vi "ATS9350_NPT_Scan.vi"(0 "Records per Buffer":u32=1000, 5 "Pt per A-line":u32=256, 7 "Total records number":u32, 9 "Numeric":dbl, 11 "Range":u32(ring)=10 items=["40 mV"=2, "100 mV"=5, "200 mV"=6, "400 mV"=7, "1 V"=10, "2 V"=11, "4 V"=12]) -> (4 "Device ID":u64)   [LabVIEW 2017]
panel:
  # "Connect proper signal to channel A before starting acquisition\n(e.g. 1Vpp 1kHz sine wave)"
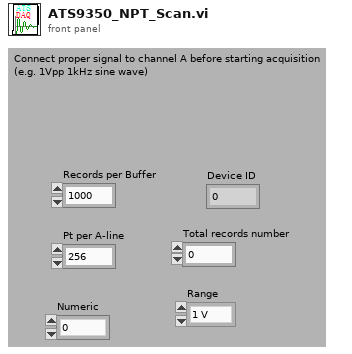
[diagram p1: front panel]
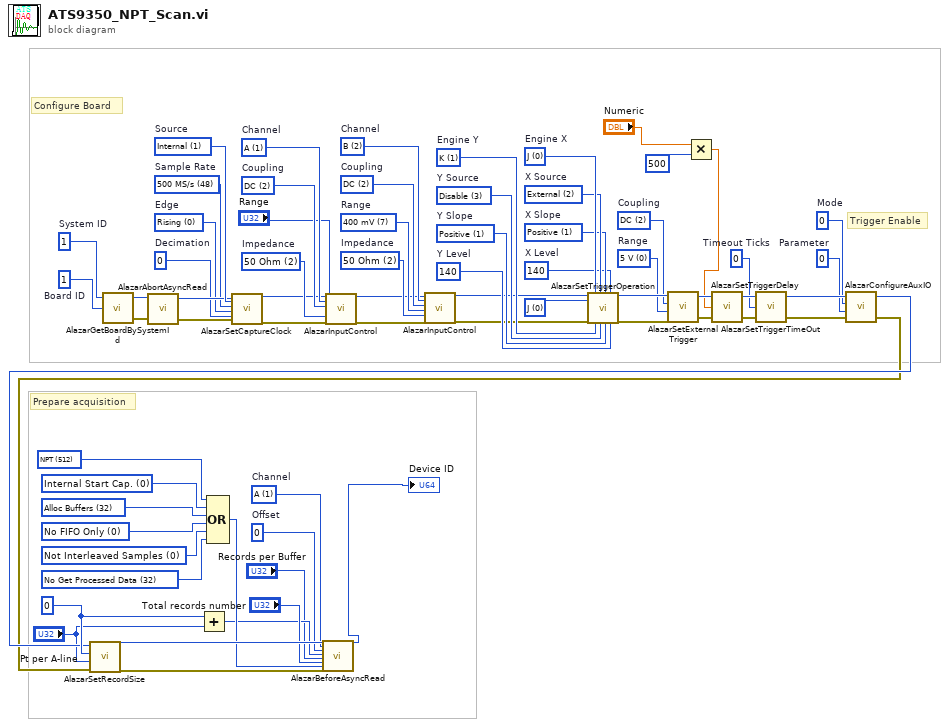
[diagram p0: block diagram]
diagram:
  w39 = u32 2 items=["50 Ohm"=2]  # Impedance
  w38 = u32 7 items=["40 mV"=2, "100 mV"=5, "200 mV"=6, "400 mV"=7, "1 V"=10, "2 V"=11, "4 V"=12]  # Range
  w40 = u32 2 items=["AC"=1, "DC"=2]  # Coupling
  w41 = u8 2 items=["A"=1, "B"=2, "C"=4, "D"=8]  # Channel
  w5 = u32 0  # Parameter
  w18 = u32 0  # Mode
  w17 = u32 0  # Timeout Ticks
  w26 = u32 0 items=["5 V", "1 V", "TTL"]  # Range
  w25 = u32 2 items=["AC"=1, "DC"=2]  # Coupling
  w29 = u32 140  # Y Level
  w30 = u32 1 items=["Positive"=1, "Negative"=2]  # Y Slope
  w31 = u32 3 items=["A", "B", "External", "Disable", "C", "D"]  # Y Source
  w33 = u32 140  # X Level
  w34 = u32 1 items=["Positive"=1, "Negative"=2]  # X Slope
  w35 = u32 2 items=["A", "B", "External", "Disable", "C", "D"]  # X Source
  w32 = u32 1 items=["J", "K"]  # Engine Y
  w36 = u32 0 items=["J", "K"]  # Engine X
  w37 = u32 0 items=["J", "K", "J OR K", "J AND K", "J XOR K", "J AND NOT K", "NOT J AND K"] ("Op.")
  w44 = u32 2 items=["50 Ohm"=2]  # Impedance
  w45 = u32 2 items=["AC"=1, "DC"=2]  # Coupling
  w46 = u8 1 items=["A"=1, "B"=2, "C"=4, "D"=8]  # Channel
  w48 = u32 0  # Decimation
  w49 = u32 0 items=["Rising", "Falling"]  # Edge
  w50 = u32 48 items=["1 kS/s"=1, "2 kS/s"=2, "5 kS/s"=4, "10 kS/s"=8, "20 kS/s"=10, "50 kS/s"=12, "100 kS/s"=14, "200 kS/s"=16, "500 kS/s"=18, "1 MS/s"=20, "2 MS/s"=24, "5 MS/s"=26, "10 MS/s"=28, "20 MS/s"=30, "50 MS/s"=34, "100 MS/s"=36, "125 MS/s"=37, "250 MS/s"=43, "500 MS/s"=48, "USER_DEF"=0]  # Sample Rate
  w52 = u32 1 items=["Internal"=1, "Fast External"=2, "Medium External"=3, "Slow External"=4, "External AC"=5, "External DC"=6, "External 10MHz"=7]  # Source
  w56 = u32 1  # Board ID
  w55 = u32 1  # System ID
  w58 = u32 0  # Offset
  w6 = u32 1 items=["A"=1, "B"=2, "A + B"=3, "C"=4, "A + C"=5, "A + B"=6, "D"=8, "A + D"=9, "B + D"=10, "C + D"=12, "A + B + C + D"=15]  # Channel
  w62 = u32 0 ("Pre-trigger Samples")
  w68 = u32 32 items=["No Get Processed Data"=32, "Get Processed Data"=8192]
  w67 = u32 0 items=["Not Interleaved Samples"=0, "Interleave Samples"=4096]
  w63 = u32 0 items=["No FIFO Only"=0, "FIFO Only"=2048]
  w66 = u32 32 items=["Alloc Buffers"=32]
  w65 = u32 0 items=["Internal Start Cap.", "External Start Cap."]
  w64 = u32 512 items=["Traditional"=0, "NPT"=512, "Continuous"=256, "Triggered Streaming"=1024]
  # "Trigger Enable"
  # "Configure Board"
  # "Prepare acquisition"
  n1 = call "AlazarGetBoardBySystemId.vi"("Board ID"=w56, "System ID"=w55) -> ("error out"=w53:errorcluster, "Handle"=w54:u64)  [unwired: 1 in, 1 out]
  n2 = call "AlazarAbortAsyncRead.vi"("Handle"=w54, "error in (no error)"=w53) -> ("Handle"=w51:u64, "error out"=w47:errorcluster)  [unwired: 1 out]
  n3 = Add(x=w62, y="Pt per A-line") -> (x+y=w10:u32)
  n4 = Compound Arithmetic op=OR(w64, w65, w66, w63, w67, w68) -> (w59:u32)
  n5 = call "AlazarSetCaptureClock.vi"("Handle"=w51, "Source"=w52, "Sample Rate"=w50, "Edge"=w49, "Decimation"=w48, "error in (no error)"=w47) -> ("Handle"=w43:u64, "error out"=w42:errorcluster)  [unwired: 11 in, 1 out]
  n6 = call "AlazarInputControl.vi"("Handle"=w43, "Channel"=w46, "Coupling"=w45, "Range"="Range", "Impedance"=w44, "error in (no error)"=w42) -> ("Handle"=w16:u64, "error out"=w15:errorcluster)  [unwired: 11 in, 1 out]
  n7 = call "AlazarInputControl.vi"("Handle"=w16, "Channel"=w41, "Coupling"=w40, "Range"=w38, "Impedance"=w39, "error in (no error)"=w15) -> ("Handle"=w13:u64, "error out"=w14:errorcluster)  [unwired: 11 in, 1 out]
  n8 = call "AlazarSetTriggerOperation.vi"("Handle"=w13, "Trigger Operation"=w37, "error in (no error)"=w14, "Trigger Engine 1"=w36, "Trigger Engine 2"=w32, "Source 1"=w35, "Source 2"=w31, "Slope 1"=w34, "Slope 2"=w30, "Level 1"=w33, "Level 2"=w29) -> ("Handle"=w28:u64, "error out"=w27:errorcluster)  [unwired: 6 in, 1 out]
  n9 = call "AlazarSetExternalTrigger.vi"("error in (no error)"=w27, "Range ID"=w26, "Coupling ID"=w25, "Handle"=w28) -> ("error out"=w23:errorcluster, "Handle"=w24:u64)  [unwired: 1 out]
  n10 = Multiply(x="Numeric", y=500) -> (x*y=w2:dbl)
  n11 = call "AlazarSetTriggerDelay.vi"("error in (no error)"=w23, "Delay"=w2, "Handle"=w24) -> ("error out"=w21:errorcluster, "Handle"=w22:u64)  [unwired: 1 out]
  n12 = call "AlazarSetTriggerTimeOut.vi"("error in (no error)"=w21, "Timeout Ticks"=w17, "Handle"=w22) -> ("error out"=w19:errorcluster, "Handle"=w20:u64)  [unwired: 1 out]
  n13 = call "AlazarConfigureAuxIO.vi"("error in (no error)"=w19, "Parameter"=w5, "Mode"=w18, "Handle"=w20) -> ("error out"=w11:errorcluster, "Handle"=w12:u64)  [unwired: 1 out]
  n14 = call "AlazarSetRecordSize.vi"("error in (no error)"=w11, "Post-trigger Samples"="Pt per A-line", "Pre-trigger Samples"=w62, "Handle"=w12) -> ("error out"=w60:errorcluster, "Handle"=w61:u64)  [unwired: 1 out]
  n15 = call "AlazarBeforeAsyncRead.vi"("Handle"=w61, "Channel Select"=w6, "Transfer Offset"=w58, "Transfer Length"=w10, "Records Per Buffer"="Records per Buffer", "Records Per Acquisition"="Total records number", "Flags"=w59, "error in (no error)"=w60) -> ("Handle"=→"Device ID":u64)  [unwired: 17 in, 2 out]
